vi "74HC112.vi"(0 "J":bool, 1 "R":bool, 2 "cp":bool, 3 "K":bool, 4 "S":bool) -> (6 "Q":bool, 7 "Q`":bool)   [LabVIEW 2018]
panel:
  # "下降沿触发的JK触发器"
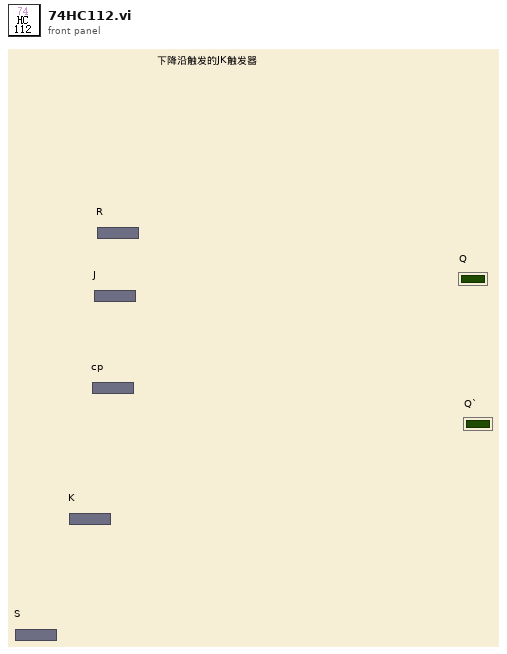
[diagram p1: front panel]
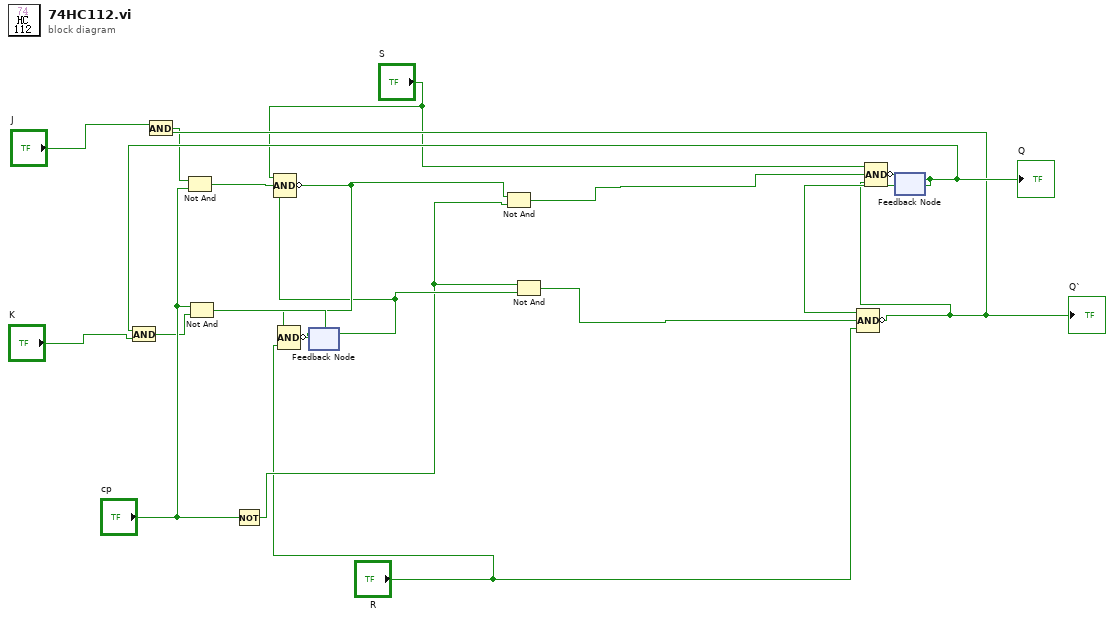
[diagram p0: block diagram]
diagram:
  n1 = Not(x="cp") -> (.not. x?=w5:bool)
  n2 = feedback #1() -> (w12:bool)  [unwired: 1 in]
  n3 = Not And(1:w12, 2:w5) -> (0:w4:bool)
  n4 = feedback #2() -> (w11:bool)  [unwired: 1 in]
  "Q" <- w11
  n5 = And(x=w11, y="K") -> (x .and. y?=w9:bool)
  n6 = Not And(1:w9, 2:"cp") -> (0:w16:bool)
  n7 = Compound Arithmetic op=AND ("复合运算")(w11, w4, "R") -> (invert w8:bool)
  "Q`" <- w8
  n8 = And(x="J", y=w8) -> (x .and. y?=w6:bool)
  n9 = Not And(1:"cp", 2:w6) -> (0:w15:bool)
  n10 = Compound Arithmetic op=AND ("复合运算")("S", w15, w12) -> (invert w14:bool)
  n11 = Compound Arithmetic op=AND ("复合运算")(w14, w16, "R") -> (invert w13:bool)
  n12 = feedback-in #1(w13) -> ()
  n13 = Not And(1:w5, 2:w14) -> (0:w3:bool)
  n14 = Compound Arithmetic op=AND ("复合运算")("S", w3, w8) -> (invert w18:bool)
  n15 = feedback-in #2(w18) -> ()
